vi "NI VeriStand - Initialize PCI Timing Engine.vi"(9 "Use External Timing In":bool, 10 "Write to  RTSI In":bool) -> (1 "Use External Timing Out":bool, 2 "Write to  RTSI Out":bool)   [LabVIEW 2010, in "NI_VS FPGA Clock Support.lvlib"]
uses:
  <userlib>/_NI VeriStand FPGA Support/NI VeriStand FPGA Clock Support/NI_VS FPGA Clock Support.lvlib
  <vilib>/eio/EIONode/EIONode.xnode
  <vilib>/rvi/eio/nirviEIOImplementation/nirviEIOImplementation.xnode
  <vilib>/rvi/eio/common/nirviEmuClasses.ctl
  <userlib>/_NI VeriStand FPGA Support/NI VeriStand FPGA Clock Support/NI VeriStand - Timing Engine Globals.vi
  <vilib>/rvi/eio/common/nirviEmuTemplateMethod_noerrors.vi
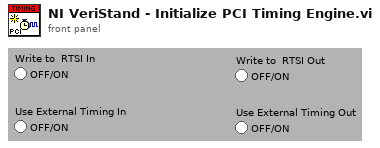
[diagram p1: front panel]
types:
  T1 = typedef "nirviEmuClasses.ctl" = enum16{"IO Read", "IO Write", "Method", "Property Read", "Property Write"}
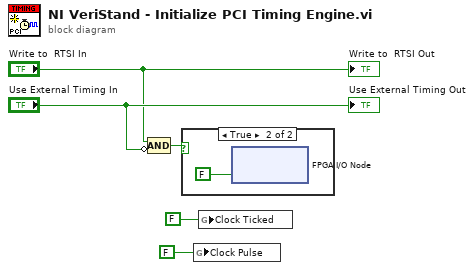
[diagram p0: block diagram]
diagram:
  n1 = Compound Arithmetic op=AND("Write to  RTSI In", invert "Use External Timing In") -> (w1:bool)
  n2 = case shown="True" w1 {
    frame False {
    }
    frame True {
      n3 = xnode "FPGA I/O Node"("RTSI0"=FALSE ("TRIG0")) -> ()  [unwired: 1 in, 1 out]
    }
  }
  n4 = global write "NI VeriStand - Timing Engine Globals.vi" "Clock Pulse"(FALSE ("Clock Ticked")) -> ()
  n5 = global write "NI VeriStand - Timing Engine Globals.vi" "Clock Ticked"(FALSE ("Clock Ticked")) -> ()
  "Write to  RTSI Out" <- "Write to  RTSI In"
  "Use External Timing Out" <- "Use External Timing In"
